vi "Pause Read Loop.vi"(8 "error in (no error)":errorcluster, 11 "Terminal in":refnum<class "Terminal.lvclass">) -> (0 "error out":errorcluster, 3 "Terminal out":refnum<class "Terminal.lvclass">)   [LabVIEW 2020, in "Terminal.lvlib" / "Terminal.lvclass"]
uses:
  Terminal.lvclass
  Terminal.lvclass/Terminal.ctl
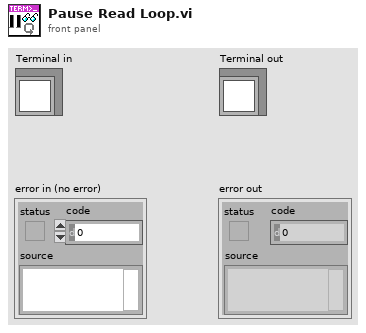
[diagram p1: front panel]
types:
  T1 = typedef "Terminal.lvlib/Terminal.lvclass/Ref Data.ctl" = cluster{"Connection":refnum<class "Connection.lvclass">, "Read Loop Running":bool, "Parse State":T2, "Terminal Options":T7, "Font Metrics":T10, "Scroll":i32, "Close Read Loop":bool, "Buffer":T11, "Pause Read Loop":bool}
  T2 = typedef "Terminal.lvlib/Terminal.lvclass/Parse State.ctl" = cluster{"Buffer State":T3, "Cursor":T4, "Attributes":T6}
  T3 = typedef "Terminal.lvlib/Terminal.lvclass/Buffer State.ctl" = cluster{"Sequence":string, "ESC":bool, "Alt Buf":bool}
  T4 = typedef "Terminal.lvlib/Terminal.lvclass/Cursor.ctl" = cluster{"Cur":T5, "Saved":T5}
  T5 = typedef "Terminal.lvlib/Terminal.lvclass/Position.ctl" = cluster{"Row":i32, "Col":i32}
  T6 = typedef "Terminal.lvlib/Text Attributes.ctl" = cluster{"FG":u32, "BG":u32, "Bold":bool, "Italic":bool, "Underline":bool, "Strike":bool, "Inverse":bool}
  T7 = typedef "Terminal.lvlib/Terminal Options.ctl" = cluster{"Implied CR with LF":bool, "Local Echo":bool, "Tab Width":i32, "Color Scheme":T8, "Default FG":T9, "Default BG":T9, "History Length":i32, "Font Face":string, "Font Size":i16, "Rows":i32, "Cols":i32}
  T8 = typedef "Terminal.lvlib/Color Scheme.ctl" = cluster{"Black":u32, "Red":u32, "Green":u32, "Yellow":u32, "Blue":u32, "Magenta":u32, "Cyan":u32, "White":u32, "Bright Black":u32, "Bright Red":u32, "Bright Green":u32, "Bright Yellow":u32, "Bright Blue":u32, "Bright Magenta":u32, "Bright Cyan":u32, "Bright White":u32}
  T9 = typedef "Terminal.lvlib/Color.ctl" = i8
  T10 = typedef "Terminal.lvlib/Terminal.lvclass/Font Metrics.ctl" = cluster{"Width":i16, "Height":i16}
  T11 = typedef "Terminal.lvlib/Buffer.ctl" = enum16{"Primary", "Alternate"}
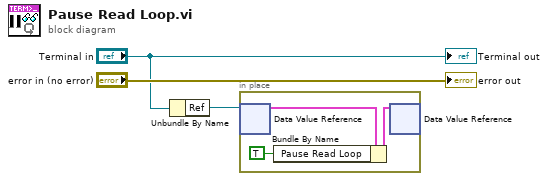
[diagram p0: block diagram]
diagram:
  n1 = Unbundle By Name("Terminal in") -> ("Ref"=w2:refnum<data-value>)
  n2 = in-place {
    n3 = in-place-dvr #1(w2) -> (w6:T1)  [unwired: 1 out]
    n4 = Bundle By Name(cluster=w6, "Pause Read Loop"=TRUE) -> (w5:T1)
    n5 = in-place-dvr #1(w5) -> ()  [unwired: 2 out]
  }
  "error out" <- "error in (no error)"
  "Terminal out" <- "Terminal in"
